vi "Main.vi"() -> ()   [LabVIEW 2020, in "MacroAssert Tests.lvlib"]
doc: "This template is for the Queued Message Handler design pattern.\n\nThe Event Handling Loop generates messages based on user interface actions.\n\nThe Message Handling Loop processes messages generated by the Event Handling Loop, or by other messages. The messages are string values, so new messages can be added easily to the Message Cases case structure in the Message Handling Loop. Each message cluster can also provide an optional value for Message Data, which is a variant that can be converted to whatever message-specific data is required."
uses:
  MacroAssert Tests.lvlib
  CTLs/UI Data.ctl
  SubVIs/Message Queue/Enqueue Message (Single).vi
  <vilib>/Utility/error.llb/Three Button Dialog (string).vi
  <vilib>/Utility/error.llb/Error Cluster From Error Code.vi
  <vilib>/ErrorRing/Error Ring.xnode
  SubVIs/Message Queue/Message Queue.lvlib
  SubVIs/User Event - Stop/User Event - Stop.lvlib
panel:
  in  "Invoke Clone Dialog":bool
  in  "Invoke Dialog":bool
  out "Display":string
  in  "Do Something Else":bool
  in  "Do Something":bool
  in  "Exit":bool
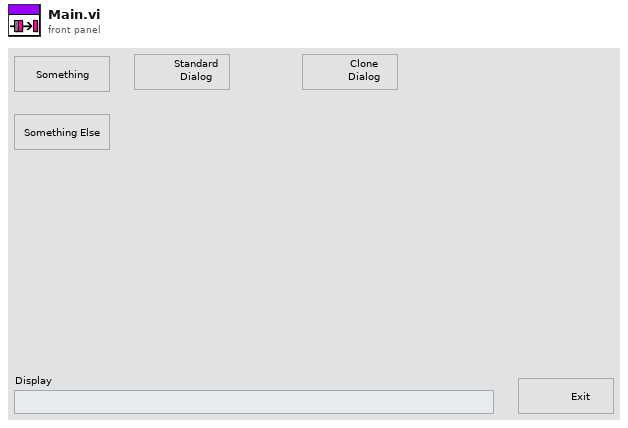
[diagram p1: front panel]
types:
  T1 = typedef "MacroAssert Tests.lvlib/UI Data.ctl" = cluster{"Boolean <Replace Me>":bool, "String <Replace Me>":string, "Numeric <Replace Me>":dbl, "Do Something Ref":refnum<vi>, "Do Something Else Ref":refnum<vi>, "Data Display Ref":refnum<vi>, "Exit Button Ref":refnum<vi>}
  T2 = typedef "MacroAssert Tests.lvlib/Message Queue.lvlib/All Message Queues.ctl" = cluster{"UI":refnum<queue>}
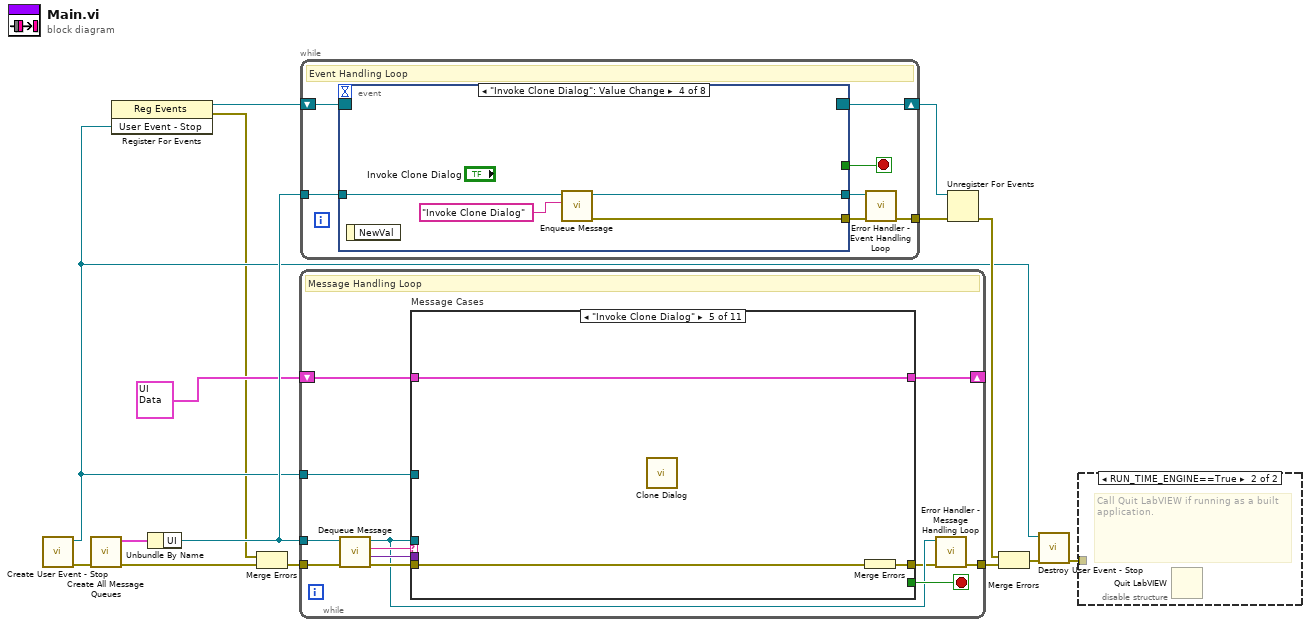
[diagram p0: block diagram]
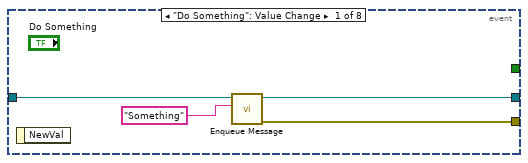
[diagram p3: hidden frame]
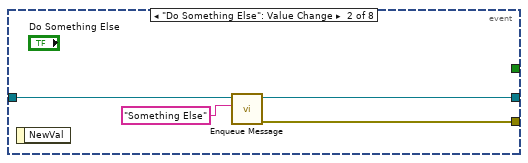
[diagram p4: hidden frame]
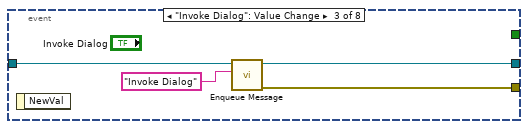
[diagram p5: hidden frame]
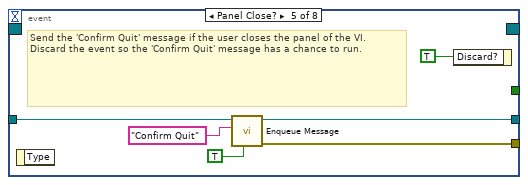
[diagram p6: hidden frame]
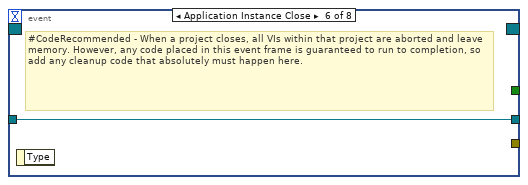
[diagram p7: hidden frame]
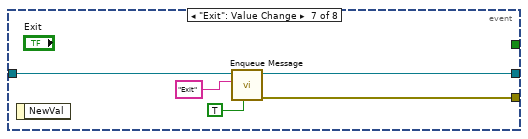
[diagram p8: hidden frame]
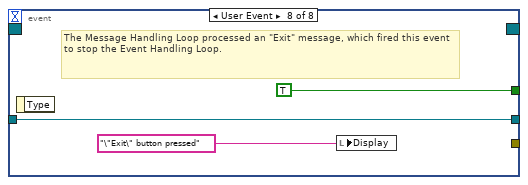
[diagram p9: hidden frame]
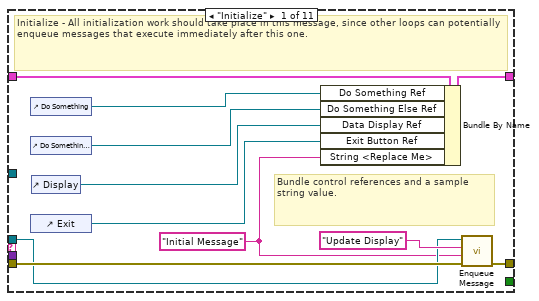
[diagram p10: hidden frame]
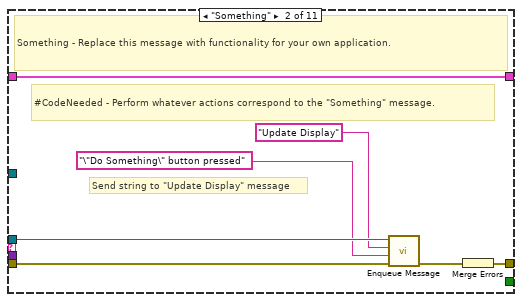
[diagram p11: hidden frame]
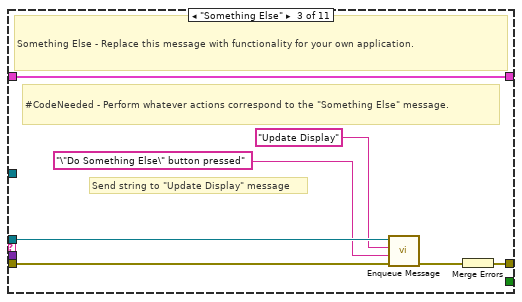
[diagram p12: hidden frame]
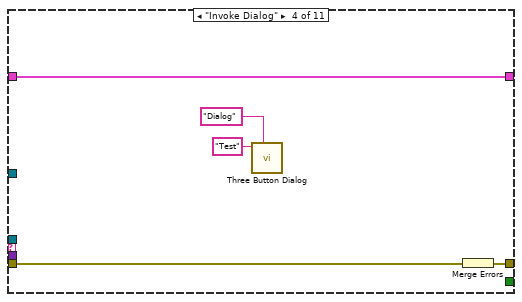
[diagram p13: hidden frame]
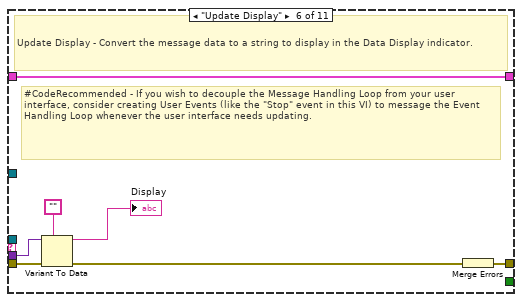
[diagram p14: hidden frame]
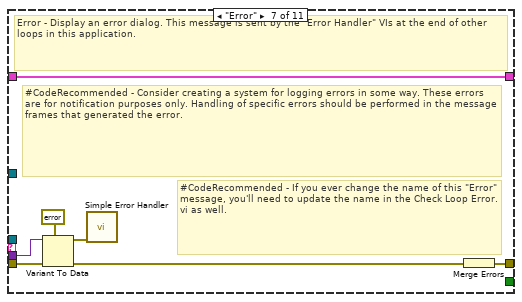
[diagram p15: hidden frame]
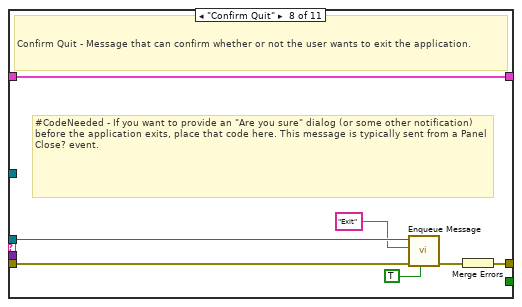
[diagram p16: hidden frame]
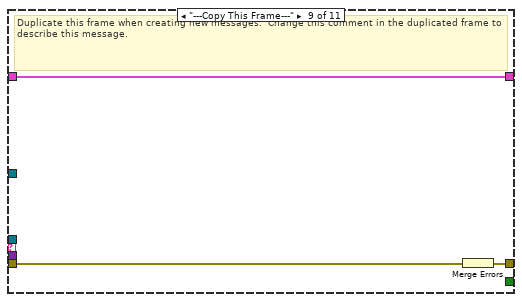
[diagram p17: hidden frame]
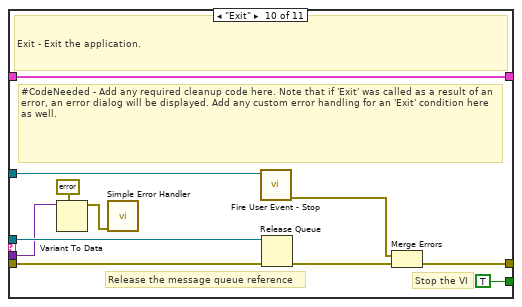
[diagram p18: hidden frame]
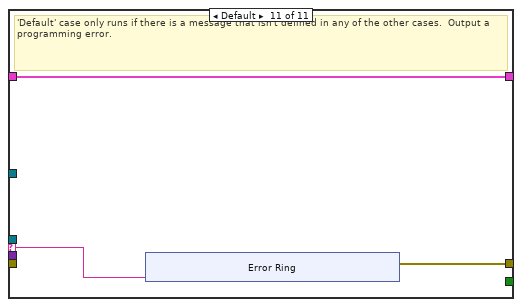
[diagram p19: hidden frame]
diagram:
  n1 = call "Create User Event - Stop.vi"() -> ("error out"=w11:errorcluster, "User Event - Stop"=w3:refnum<user-event>)  [unwired: 10 in]
  n2 = call "Create All Message Queues.vi"("error in (no error)"=w11) -> ("error out"=w15:errorcluster, "Message Queues out"=w14:T2)  [unwired: 9 in]
  n3 = register-events(w3) -> (reference out=w4:refnum<event-registration>, error out=w1:errorcluster)  [unwired: 2 in]
  n4 = Unbundle By Name(w14) -> ("UI"=w12:refnum<queue>)
  n5 = Merge Errors(w1, w15) -> (w2:errorcluster)
  n6 = while {
    tunnel: w12 -> [w19]
    shift-right: [w26] -> _
    shift-left: T1 {"Boolean <Replace Me>"=FALSE, "String <Replace Me>"="", "Numeric <Replace Me>"=0.0, "Do Something Ref"=refnum, "Do Something Else Ref"=refnum, "Data Display Ref"=refnum, "Exit Button Ref"=refnum} ("Data Cluster") -> [w27]
    tunnel: w3 -> [w24]
    tunnel: w2 -> [w23]
    tunnel: [w17] -> w13
    stop <- w25 stop-if-true
    # "Message Handling Loop"
    n7 = call "Dequeue Message.vi"("error in (no error)"=w23, "Message Queue"=w19) -> ("error out"=w22:errorcluster, "Message Data"=w20:variant, "Message"=w21:string, "dup Message Queue"=w18:refnum<queue>)  [unwired: 6 in]
    n8 = case "Message Cases" shown="\"Invoke Clone Dialog\"" w21 {
      selector: w21 -> [_ _ _ _ _ _ _ _ _ _ w96]
      tunnel: w18 -> [w29 w41 w48 _ _ _ _ w77 _ w95 _]
      tunnel: w22 -> [w37 w43 w50 w54 w58 w65 w74 w81 w84 w88 _]
      tunnel: [w38 w44 w51 w56 w59 w66 w68 w79 w82 w91 w97] -> w16
      tunnel: w27 -> [w36 w45 w52 w57 w60 w67 w73 w80 w83 w94 w98]
      tunnel: [w35 w45 w52 w57 w60 w67 w73 w80 w83 w94 w98] -> w26
      tunnel: [_ _ _ _ _ _ _ _ _ TRUE _] -> w25
      tunnel: w20 -> [_ _ _ _ _ w64 w72 _ _ w85 _]
      tunnel: w24 -> [_ _ _ _ _ _ _ _ _ w90 _]
      frame "Initialize" {
        w28 = "Initial Message" ("Initial Message")
        # "Bundle control references and a sample string value."
        # "Initialize - All initialization work should take place in this message, since other loops can potentially enqueue messages that execute immediately after this one."
        n9 = control-ref of="Do Something"() -> (w34:refnum<vi>)
        n10 = control-ref of="Do Something Else"() -> (w33:refnum<vi>)
        n11 = control-ref of="Exit"() -> (w31:refnum<vi>)
        n12 = control-ref of="Display"() -> (w32:refnum<vi>)
        n13 = Bundle By Name(cluster=w36, "Do Something Ref"=w34, "Do Something Else Ref"=w33, "Data Display Ref"=w32, "Exit Button Ref"=w31, "String <Replace Me>"=w28) -> (w35:T1)
        n14 = call-poly "Enqueue Message.vi"("error in (no error)"=w37, "Message Data"=w28, "Message"="Update Display", "Message Queue"=w29) -> ("error out"=w38:errorcluster)  [unwired: 6 in, 1 out]
      }
      frame "Something" {
        # "Send string to \"Update Display\" message"
        # "#CodeNeeded - Perform whatever actions correspond to the \"Something\" message."
        # "Something - Replace this message with functionality for your own application."
        n15 = call-poly "Enqueue Message.vi"("error in (no error)"=w43, "Message Data"="\"Do Something\" button pressed" ("\"Do Something\" button pressed"), "Message"="Update Display", "Message Queue"=w41) -> ("error out"=w42:errorcluster)  [unwired: 6 in, 1 out]
        n16 = Merge Errors(w42) -> (w44:errorcluster)
      }
      frame "Something Else" {
        # "Send string to \"Update Display\" message"
        # "#CodeNeeded - Perform whatever actions correspond to the \"Something Else\" message."
        # "Something Else - Replace this message with functionality for your own application."
        n17 = call-poly "Enqueue Message.vi"("error in (no error)"=w50, "Message Data"="\"Do Something Else\" button pressed" ("\"Do Something Else\" button pressed"), "Message"="Update Display", "Message Queue"=w48) -> ("error out"=w49:errorcluster)  [unwired: 6 in, 1 out]
        n18 = Merge Errors(w49) -> (w51:errorcluster)
      }
      frame "Invoke Dialog" {
        n19 = call-poly <vilib>:"Three Button Dialog.vi"("Window Title (\"\")"="Dialog" ("Window Title (\"\")"), "message"="Test") -> ()  [unwired: 9 in, 1 out]
        n20 = Merge Errors(w54) -> (w56:errorcluster)
      }
      frame "Invoke Clone Dialog" {
        n21 = call "Clone Dialog.vi"() -> ()  [unwired: 12 in]
        n22 = Merge Errors(w58) -> (w59:errorcluster)
      }
      frame "Update Display" {
        # "#CodeRecommended - If you wish to decouple the Message Handling Loop from your user interface, consider creating User Events (like the \"Stop\" event in this VI) to message the Event Handling Loop whenever the user interface needs updating."
        # "Update Display - Convert the message data to a string to display in the Data Display indicator."
        n23 = Variant To Data(error in=w65, type="", Variant=w64) -> (data=→"Display":string, error out=w62:errorcluster)
        n24 = Merge Errors(w62) -> (w66:errorcluster)
      }
      frame "Error" {
        # "#CodeRecommended - If you ever change the name of this \"Error\" message, you'll need to update the name in the Check Loop Error.vi as well."
        # "#CodeRecommended - Consider creating a system for logging errors in some way. These errors are for notification purposes only. Handling of specific errors should be performed in the message frames that generated the error."
        # "Error - Display an error dialog. This message is sent by the \"Error Handler\" VIs at the end of other loops in this application."
        n25 = Variant To Data(error in=w74, type=errorcluster {"status"=FALSE, "code"=0, "source"=""} ("error constant"), Variant=w72) -> (data=w70:errorcluster, error out=w69:errorcluster)
        n26 = call <vilib>:"Simple Error Handler.vi"("error in (no error)"=w70) -> ()  [unwired: 4 in, 5 out]
        n27 = Merge Errors(w69) -> (w68:errorcluster)
      }
      frame "Confirm Quit" {
        # "#CodeNeeded - If you want to provide an \"Are you sure\" dialog (or some other notification) before the application exits, place that code here. This message is typically sent from a Panel Close? event."
        # "Confirm Quit - Message that can confirm whether or not the user wants to exit the application."
        n28 = call-poly "Enqueue Message.vi"("Priority Message? (F)"=TRUE, "error in (no error)"=w81, "Message"="Exit", "Message Queue"=w77) -> ("error out"=w78:errorcluster)  [unwired: 6 in, 1 out]
        n29 = Merge Errors(w78) -> (w79:errorcluster)
      }
      frame "---Copy This Frame---" {
        # "Duplicate this frame when creating new messages.  Change this comment in the duplicated frame to describe this message."
        n30 = Merge Errors(w84) -> (w82:errorcluster)
      }
      frame "Exit" {
        # "Stop the VI"
        # "Release the message queue reference"
        # "#CodeNeeded - Add any required cleanup code here. Note that if 'Exit' was called as a result of an error, an error dialog will be displayed. Add any custom error handling for an 'Exit' condition here as well."
        # "Exit - Exit the application."
        n31 = Variant To Data(type=errorcluster {"status"=FALSE, "code"=0, "source"=""} ("error constant"), Variant=w85) -> (data=w86:errorcluster)  [unwired: 1 in, 1 out]
        n32 = call <vilib>:"Simple Error Handler.vi"("error in (no error)"=w86) -> ()  [unwired: 4 in, 5 out]
        n33 = call "Fire User Event - Stop.vi"("User Event - Stop"=w90) -> ("error out"=w89:errorcluster)  [unwired: 10 in]
        n34 = Release Queue(queue=w95, error in (no error)=w88) -> (error out=w92:errorcluster)  [unwired: 1 in, 2 out]
        n35 = Merge Errors(w89, w92) -> (w91:errorcluster)
      }
      frame Default {
        # "'Default' case only runs if there is a message that isn't defined in any of the other cases.  Output a programming error."
        n36 = xnode "Error Ring"("parameter 0"=w96) -> ("error out"=w97:errorcluster)
      }
    }
    n37 = call "Error Handler - Message Handling Loop.vi"("error in (no error)"=w16, "Message Queue"=w18) -> ("dup error in"=w17:errorcluster)  [unwired: 8 in, 1 out]
  }
  n38 = while {
    tunnel: w12 -> [w112]
    shift-right: [w110] -> w8
    shift-left: w4 -> [w111]
    tunnel: [w106] -> w5
    stop <- w108 stop-if-true
    # "Event Handling Loop"
    n39 = event shown="[3] \"Invoke Clone Dialog\": Value Change" {
      selector: w111 -> [_ _ _ _ _ _ _ _]
      dyn-events: [_ _ _ _ _ _ _ _] -> w110
      timeout: _ -> [_ _ _ _ _ _ _ _]
      tunnel: [_ _ _ _ _ _ _ TRUE ("Discard?")] -> w108
      tunnel: w112 -> [w116 w120 w124 w128 w133 w135 w140 w143]
      tunnel: [w113 w117 w121 w125 w132 _ w139 _] -> w109
      tunnel: [w115 w119 w123 w127 w131 w135 w138 w143] -> w107
      event "Do Something": Value Change {
        n40 = event-data() -> ()  [unwired: 1 in, 1 out]
        n41 = call-poly "Enqueue Message.vi"("Message"="Something", "Message Queue"=w116) -> ("error out"=w113:errorcluster, "dup Message Queue"=w115:refnum<queue>)  [unwired: 8 in]
      }
      event "Do Something Else": Value Change {
        n42 = event-data() -> ()  [unwired: 1 in, 1 out]
        n43 = call-poly "Enqueue Message.vi"("Message"="Something Else", "Message Queue"=w120) -> ("error out"=w117:errorcluster, "dup Message Queue"=w119:refnum<queue>)  [unwired: 8 in]
      }
      event "Invoke Dialog": Value Change {
        n44 = event-data() -> ()  [unwired: 1 in, 1 out]
        n45 = call-poly "Enqueue Message.vi"("Message"="Invoke Dialog", "Message Queue"=w124) -> ("error out"=w121:errorcluster, "dup Message Queue"=w123:refnum<queue>)  [unwired: 8 in]
      }
      event "Invoke Clone Dialog": Value Change {
        n46 = event-data() -> ()  [unwired: 1 in, 1 out]
        n47 = call-poly "Enqueue Message.vi"("Message"="Invoke Clone Dialog", "Message Queue"=w128) -> ("error out"=w125:errorcluster, "dup Message Queue"=w127:refnum<queue>)  [unwired: 8 in]
      }
      event Panel Close? {
        # "Send the 'Confirm Quit' message if the user closes the panel of the VI. Discard the event so the 'Confirm Quit' message has a chance to run."
        n48 = event-data() -> ()  [unwired: 1 in, 1 out]
        n49 = call-poly "Enqueue Message.vi"("Priority Message? (F)"=TRUE, "Message"="Confirm Quit", "Message Queue"=w133) -> ("error out"=w132:errorcluster, "dup Message Queue"=w131:refnum<queue>)  [unwired: 7 in]
        n50 = event-data("Discard?"=TRUE) -> ()  [unwired: 1 in, 1 out]
      }
      event Application Instance Close {
        # "#CodeRecommended - When a project closes, all VIs within that project are aborted and leave memory. However, any code placed in this event frame is guaranteed to run to completion, so add any cleanup code that absolutely must happen here."
        n51 = event-data() -> ()  [unwired: 1 in, 1 out]
      }
      event "Exit": Value Change {
        n52 = event-data() -> ()  [unwired: 1 in, 1 out]
        n53 = call-poly "Enqueue Message.vi"("Priority Message? (F)"=TRUE, "Message"="Exit", "Message Queue"=w140) -> ("error out"=w139:errorcluster, "dup Message Queue"=w138:refnum<queue>)  [unwired: 7 in]
      }
      event User Event {
        # "The Message Handling Loop processed an \"Exit\" message, which fired this event to stop the Event Handling Loop."
        n54 = event-data() -> ()  [unwired: 1 in, 1 out]
        n55 = local write "Display"("\"Exit\" button pressed" ("VI Stopped")) -> ()
      }
    }
    n56 = call "Error Handler - Event Handling Loop.vi"("error in (no error)"=w109, "Message Queue"=w107) -> ("dup error in"=w106:errorcluster)  [unwired: 8 in, 1 out]
  }
  n57 = Unregister For Events(event registration refnum=w8, error in=w5) -> (error out=w9:errorcluster)
  n58 = Merge Errors(w9, w13) -> (w10:errorcluster)
  n59 = call "Destroy User Event - Stop.vi"("error in (no error)"=w10, "User Event - Stop"=w3) -> ("error out"=w6:errorcluster)  [unwired: 9 in]
  n60 = disable-structure shown="RUN_TIME_ENGINE==True" {
    disable-tunnel: w6 -> [_ _]
    frame condition #0 (active) {
    }
    frame condition #1 {
      # "Call Quit LabVIEW if running as a built application."
      n61 = Quit LabVIEW() -> ()  [unwired: 1 in]
    }
  }
